vi "Swerve Motor Back Left new.vi"(2 "Speed command":dbl, 3 "Direction command (deg)":dbl) -> ()   [LabVIEW 2018]
panel:
  out "Flip motors?":bool
  out "New Position":dbl
  in  "Offset":dbl
  out "Swerve Y N":bool
  out "Degres To Travel":dbl
  out "Better Angle 2":dbl(knob)=41.7137932364482 scale=0.0..360.0
  out "Veloicity":dbl
  in  "Back Left Angle":dbl
  # "VI inputs"
  # "Intermediate values"
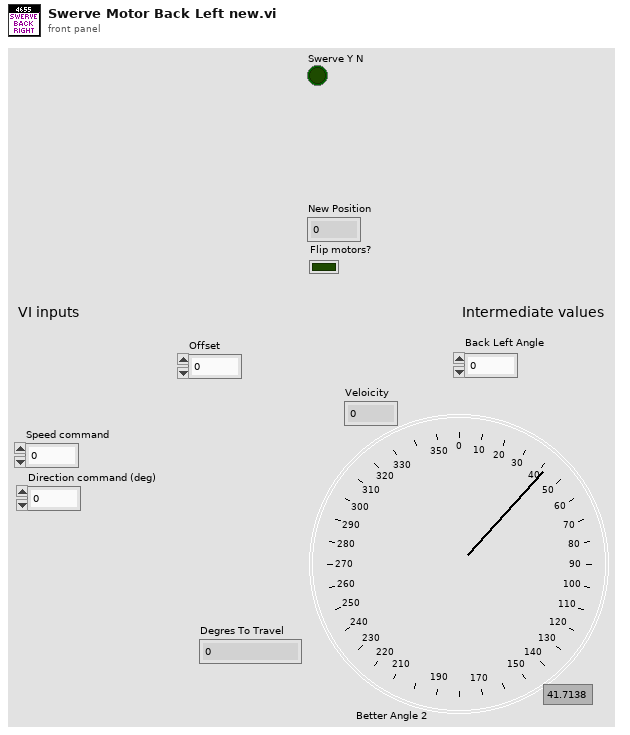
[diagram p1: front panel]
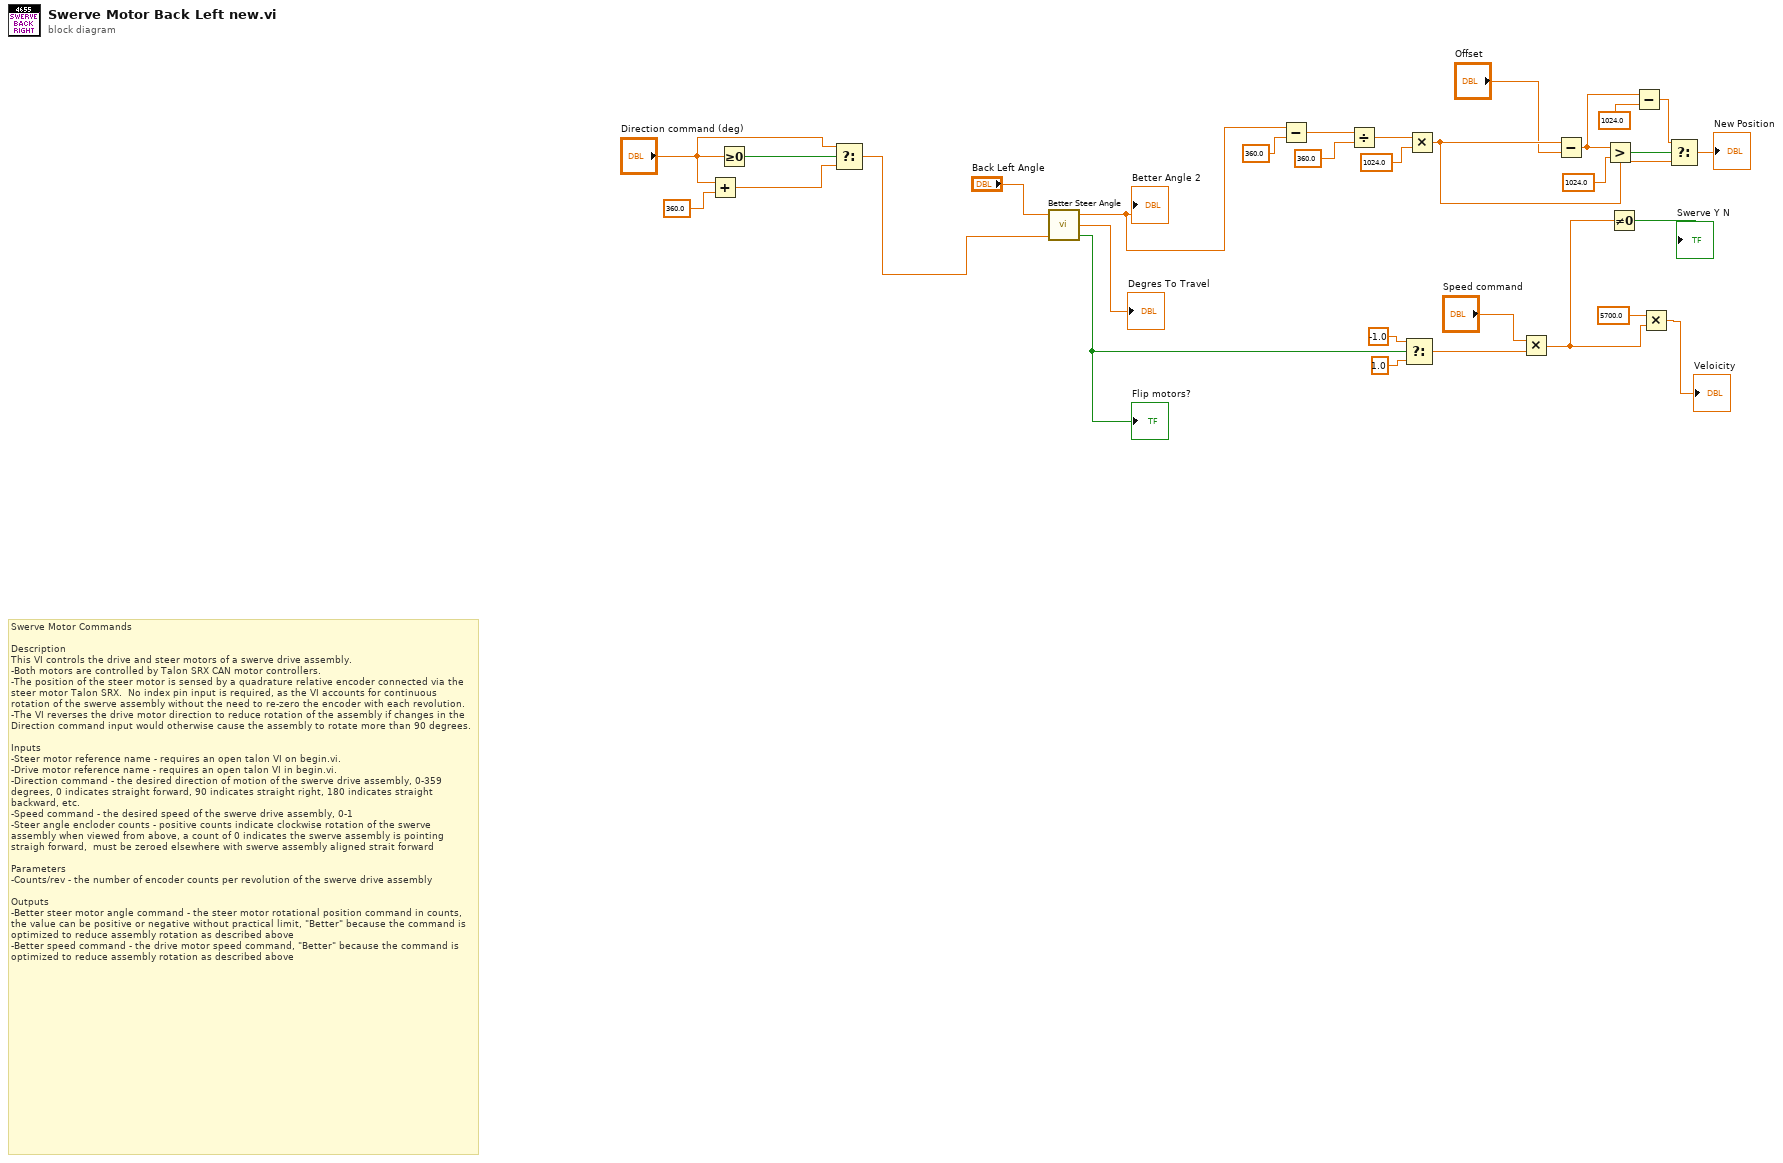
[diagram p0: block diagram]
diagram:
  # "Swerve Motor Commands\n\nDescription\nThis VI controls the drive and steer motors of a swerve drive assembly.  \n-Both motors are controlled by Talon SRX CAN motor controllers.  \n-The position of the steer motor is sensed by a quadrature relative encoder connected via the steer motor Talon SRX.  No index pin input is required, as the VI accounts for continuous rotation of the swerve assembly without the need to re-zero the encoder with each revolution.\n-The VI reverses the drive motor direction to reduce rotation of the assembly if changes in the Direction command input would otherwise cause the assembly to rotate more than 90 degrees.\n\nInputs\n-Steer motor reference name - requires an open talon VI on begin.vi.\n-Drive motor reference name - requires an open talon VI in begin.vi.\n-Direction command - the desired direction of motion of the swerve drive assembly, 0-359 degrees, 0 indicates straight forward, 90 indicates straight right, 180 indicates straight backward, etc.\n-Speed command - the desired speed of the swerve drive assembly, 0-1\n-Steer angle encloder counts - positive counts indicate clockwise rotation of the swerve assembly when viewed from above, a count of 0 indicates the swerve assembly is pointing straigh forward,  must be zeroed elsewhere with swerve assembly aligned strait forward\n\nParameters\n-Counts/rev - the number of encoder counts per revolution of the swerve drive assembly\n\nOutputs\n-Better steer motor angle command - the steer motor rotational position command in counts, the value can be positive or negative without practical limit, \"Better\" because the command is optimized to reduce assembly rotation as described above\n-Better speed command - the drive motor speed command, \"Better\" because the command is optimized to reduce assembly rotation as described above"
  n1 = Add(x="Direction command (deg)", y=360.0) -> (x+y=w18:dbl)
  n2 = Greater Or Equal To 0?(x="Direction command (deg)") -> (x >= 0?=w20:bool)
  n3 = Select(t="Direction command (deg)", s=w20, f=w18) -> (s? t:f=w3:dbl)
  n4 = call "Better Steer Angle.vi"("Set Point"=w3, "Current Angle"="Back Left Angle") -> ("Flip motors?"=w1:bool, "Degres To Travel"=→"Degres To Travel":dbl, "Better Angle"=w2:dbl)  [unwired: 1 in]
  "Better Angle 2" <- w2
  "Flip motors?" <- w1
  n5 = Subtract(x=w2, y=360.0) -> (x-y=w15:dbl)
  n6 = Divide(x=w15, y=360.0) -> (x/y=w24:dbl)
  n7 = Select(t=-1.0, s=w1, f=1.0) -> (s? t:f=w28:dbl)
  n8 = Multiply(x=w24, y=1024.0 ("x*y")) -> (x*y=w9:dbl)
  n9 = Multiply(x="Speed command", y=w28) -> (x*y=w21:dbl)
  n10 = Subtract(x=w9, y="Offset") -> (x-y=w12:dbl)
  n11 = Greater?(x=w12, y=1024.0) -> (0:w13:bool)
  n12 = Not Equal To 0?(x=w21) -> (x != 0?=→"Swerve Y N":bool)
  n13 = Subtract(x=w12, y=1024.0) -> (x-y=w10:dbl)
  n14 = Multiply(x=5700.0, y=w21) -> (x*y=→"Veloicity":dbl)
  n15 = Select(t=w10, s=w13, f=w9) -> (s? t:f=→"New Position":dbl)
